vi "test_FindProjects.vi"() -> (3 "Pass?":bool)   [LabVIEW 2020, in "Tests.SolutionBuilder.lvlib"]
uses:
  Tests.SolutionBuilder.lvlib
  SolutionBuilder/SolutionBuilder.lvclass
panel:
  out "test results":u32 format="%07b"
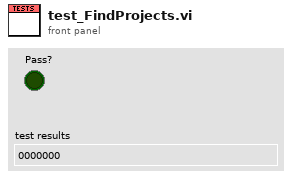
[diagram p1: front panel]
types:
  T1 = typedef "SolutionBuilder.lvlib/SolutionBuilder.lvclass/ProjectItemMap.ctl" = map{path, refnum<class "ProjectItem.lvclass">[]}
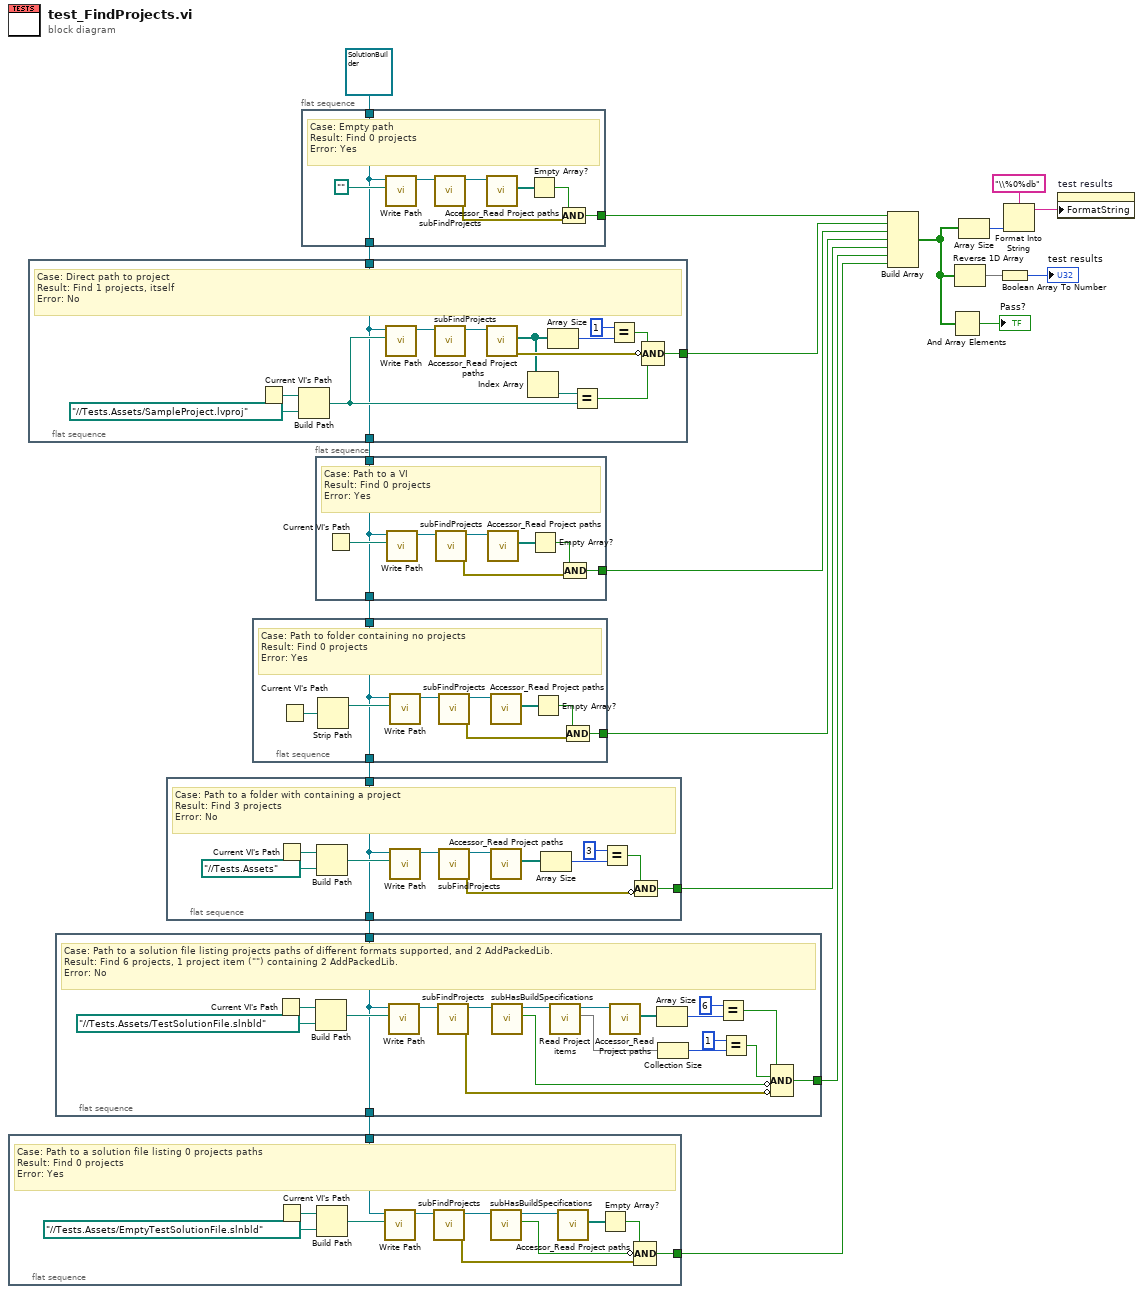
[diagram p0: block diagram]
diagram:
  n1 = flat-sequence {
    tunnel: [w26] -> w8
    tunnel: w2 -> [w25]
    frame #0 {
      # "Case: Path to a solution file listing 0 projects paths\nResult: Find 0 projects\nError: Yes"
      n2 = Current VI's Path() -> (path=w28:path)
      n3 = Build Path(base path=w28, name or relative path=path "../../Tests.Assets/EmptyTestSolutionFile.slnbld" ("Path")) -> (appended path=w27:path)
      n4 = call-dynamic "Write Path.vi"("Path"=w27, "SolutionBuilder in"=w25) -> ("SolutionBuilder out"=w30:refnum<class "SolutionBuilder.lvclass">)  [unwired: 9 in]
      n5 = call "subFindProjects.vi"("SolutionBuilder in"=w30) -> ("error out"=w31:errorcluster, "SolutionBuilder out"=w24:refnum<class "SolutionBuilder.lvclass">)  [unwired: 9 in]
      n6 = call "subHasBuildSpecifications.vi"("SolutionBuilder in"=w24) -> ("Has specs?"=w22:bool, "SolutionBuilder out"=w23:refnum<class "SolutionBuilder.lvclass">)  [unwired: 8 in, 1 out]
      n7 = call "Accessor_Read Project paths.vi"("SolutionBuilder in"=w23) -> ("Project paths"=w32:path[])  [unwired: 8 in, 2 out]
      n8 = Empty Array?(array=w32) -> (empty?=w33:bool)
      n9 = Compound Arithmetic op=AND(w33, invert w22, w31) -> (w26:bool)
    }
  }
  n10 = flat-sequence {
    tunnel: [w39] -> w14
    tunnel: w7 -> [w34]
    tunnel: [w34] -> w6
    frame #0 {
      # "Case: Direct path to project\nResult: Find 1 projects, itself\nError: No"
      n11 = Current VI's Path() -> (path=w45:path)
      n12 = Build Path(base path=w45, name or relative path=path "../../Tests.Assets/SampleProject.lvproj" ("Path")) -> (appended path=w36:path)
      n13 = call-dynamic "Write Path.vi"("Path"=w36, "SolutionBuilder in"=w34) -> ("SolutionBuilder out"=w47:refnum<class "SolutionBuilder.lvclass">)  [unwired: 9 in]
      n14 = call "subFindProjects.vi"("SolutionBuilder in"=w47) -> ("SolutionBuilder out"=w46:refnum<class "SolutionBuilder.lvclass">)  [unwired: 9 in, 1 out]
      n15 = call "Accessor_Read Project paths.vi"("SolutionBuilder in"=w46) -> ("error out"=w40:errorcluster, "Project paths"=w38:path[])  [unwired: 8 in, 1 out]
      n16 = Index Array(array=w38) -> (element=w37:path)  [unwired: 1 in]
      n17 = Array Size(array=w38) -> (size(s)=w43:i32)
      n18 = Equal?(x=w37, y=w36) -> (x = y?=w35:bool)
      n19 = Equal?(x=1, y=w43) -> (x = y?=w41:bool)
      n20 = Compound Arithmetic op=AND(w41, invert w40, w35) -> (w39:bool)
    }
  }
  n21 = flat-sequence {
    tunnel: [w60] -> w10
    tunnel: w3 -> [w56]
    tunnel: [w56] -> w2
    frame #0 {
      # "Case: Path to a solution file listing projects paths of different formats supported, and 2 AddPackedLib. \nResult: Find 6 projects, 1 project item (\"\") containing 2 AddPackedLib.\nError: No"
      n22 = Current VI's Path() -> (path=w65:path)
      n23 = Build Path(base path=w65, name or relative path=path "../../Tests.Assets/TestSolutionFile.slnbld" ("Path")) -> (appended path=w57:path)
      n24 = call-dynamic "Write Path.vi"("Path"=w57, "SolutionBuilder in"=w56) -> ("SolutionBuilder out"=w66:refnum<class "SolutionBuilder.lvclass">)  [unwired: 9 in]
      n25 = call "subFindProjects.vi"("SolutionBuilder in"=w66) -> ("error out"=w59:errorcluster, "SolutionBuilder out"=w50:refnum<class "SolutionBuilder.lvclass">)  [unwired: 9 in]
      n26 = call "subHasBuildSpecifications.vi"("SolutionBuilder in"=w50) -> ("Has specs?"=w48:bool, "SolutionBuilder out"=w49:refnum<class "SolutionBuilder.lvclass">)  [unwired: 8 in, 1 out]
      n27 = call-dynamic "Read Project items.vi"("SolutionBuilder in"=w49) -> ("Project items"=w52:T1, "SolutionBuilder out"=w55:refnum<class "SolutionBuilder.lvclass">)  [unwired: 9 in]
      n28 = call "Accessor_Read Project paths.vi"("SolutionBuilder in"=w55) -> ("Project paths"=w58:path[])  [unwired: 8 in, 2 out]
      n29 = Array Size(array=w58) -> (size(s)=w63:i32)
      n30 = Collection Size(1:w52) -> (0:w53:i32)
      n31 = Equal?(x=6, y=w63) -> (x = y?=w61:bool)
      n32 = Equal?(x=1, y=w53) -> (x = y?=w51:bool)
      n33 = Compound Arithmetic op=AND(w61, w51, invert w48, invert w59) -> (w60:bool)
    }
  }
  n34 = flat-sequence {
    tunnel: [w69] -> w11
    tunnel: w4 -> [w67]
    tunnel: [w67] -> w3
    frame #0 {
      # "Case: Path to a folder with containing a project\nResult: Find 3 projects\nError: No"
      n35 = Current VI's Path() -> (path=w72:path)
      n36 = Build Path(base path=w72, name or relative path=path "../../Tests.Assets" ("Path")) -> (appended path=w78:path)
      n37 = call-dynamic "Write Path.vi"("Path"=w78, "SolutionBuilder in"=w67) -> ("SolutionBuilder out"=w70:refnum<class "SolutionBuilder.lvclass">)  [unwired: 9 in]
      n38 = call "subFindProjects.vi"("SolutionBuilder in"=w70) -> ("error out"=w68:errorcluster, "SolutionBuilder out"=w71:refnum<class "SolutionBuilder.lvclass">)  [unwired: 9 in]
      n39 = call "Accessor_Read Project paths.vi"("SolutionBuilder in"=w71) -> ("Project paths"=w77:path[])  [unwired: 8 in, 2 out]
      n40 = Array Size(array=w77) -> (size(s)=w74:i32)
      n41 = Equal?(x=3, y=w74) -> (x = y?=w76:bool)
      n42 = Compound Arithmetic op=AND(w76, invert w68) -> (w69:bool)
    }
  }
  n43 = flat-sequence {
    tunnel: [w80] -> w12
    tunnel: w5 -> [w79]
    tunnel: [w79] -> w4
    frame #0 {
      # "Case: Path to folder containing no projects\nResult: Find 0 projects\nError: Yes"
      n44 = Current VI's Path() -> (path=w82:path)
      n45 = Strip Path(path=w82) -> (stripped path=w81:path)  [unwired: 1 out]
      n46 = call-dynamic "Write Path.vi"("Path"=w81, "SolutionBuilder in"=w79) -> ("SolutionBuilder out"=w87:refnum<class "SolutionBuilder.lvclass">)  [unwired: 9 in]
      n47 = call "subFindProjects.vi"("SolutionBuilder in"=w87) -> ("error out"=w85:errorcluster, "SolutionBuilder out"=w86:refnum<class "SolutionBuilder.lvclass">)  [unwired: 9 in]
      n48 = call "Accessor_Read Project paths.vi"("SolutionBuilder in"=w86) -> ("Project paths"=w84:path[])  [unwired: 8 in, 2 out]
      n49 = Empty Array?(array=w84) -> (empty?=w83:bool)
      n50 = Compound Arithmetic op=AND(w83, w85) -> (w80:bool)
    }
  }
  n51 = flat-sequence {
    tunnel: [w90] -> w15
    tunnel: refnum<class "SolutionBuilder.lvclass"> refnum ("SolutionBuilder in") -> [w88]
    tunnel: [w88] -> w7
    frame #0 {
      # "Case: Empty path\nResult: Find 0 projects\nError: Yes"
      n52 = call-dynamic "Write Path.vi"("Path"=path "", "SolutionBuilder in"=w88) -> ("SolutionBuilder out"=w95:refnum<class "SolutionBuilder.lvclass">)  [unwired: 9 in]
      n53 = call "subFindProjects.vi"("SolutionBuilder in"=w95) -> ("error out"=w93:errorcluster, "SolutionBuilder out"=w94:refnum<class "SolutionBuilder.lvclass">)  [unwired: 9 in]
      n54 = call "Accessor_Read Project paths.vi"("SolutionBuilder in"=w94) -> ("Project paths"=w92:path[])  [unwired: 8 in, 2 out]
      n55 = Empty Array?(array=w92) -> (empty?=w91:bool)
      n56 = Compound Arithmetic op=AND(w91, w93) -> (w90:bool)
    }
  }
  n57 = flat-sequence {
    tunnel: [w97] -> w13
    tunnel: w6 -> [w96]
    tunnel: [w96] -> w5
    frame #0 {
      # "Case: Path to a VI\nResult: Find 0 projects\nError: Yes"
      n58 = Current VI's Path() -> (path=w98:path)
      n59 = call-dynamic "Write Path.vi"("Path"=w98, "SolutionBuilder in"=w96) -> ("SolutionBuilder out"=w99:refnum<class "SolutionBuilder.lvclass">)  [unwired: 9 in]
      n60 = call "subFindProjects.vi"("SolutionBuilder in"=w99) -> ("error out"=w101:errorcluster, "SolutionBuilder out"=w100:refnum<class "SolutionBuilder.lvclass">)  [unwired: 9 in]
      n61 = call "Accessor_Read Project paths.vi"("SolutionBuilder in"=w100) -> ("Project paths"=w102:path[])  [unwired: 8 in, 2 out]
      n62 = Empty Array?(array=w102) -> (empty?=w103:bool)
      n63 = Compound Arithmetic op=AND(w103, w101) -> (w97:bool)
    }
  }
  n64 = Build Array(w15, w14, w13, w12, w11, w10, w8) -> (w19:bool[])
  n65 = And Array Elements(Boolean array=w19) -> (logical AND=→"Pass?":bool)
  n66 = Reverse 1D Array(array=w19) -> (reversed array=w1:bool[])
  n67 = Array Size(array=w19) -> (size(s)=w17:i32)
  n68 = Boolean Array To Number(Boolean array=w1) -> (number=→"test results":u32)
  n69 = Format Into String(format string="\\%0%db", w17) -> (resulting string=w16:string)  [unwired: 2 in, 1 out]
  n70 = property on="test results" class="DigNum (strict)"("FormatString"=w16) -> ()  [unwired: 2 in, 2 out]
